vi "Init Test Group.vi"(8 "error in (no error)":errorcluster, 11 "Servo MSMT in":refnum<class "Servo MSMT.lvclass">) -> (0 "error out":errorcluster, 3 "Servo MSMT out":refnum<class "Servo MSMT.lvclass">)   [LabVIEW 2018, in "Servo MSMT.lvlib" / "Servo MSMT.lvclass"]
uses:
  Servo MSMT.lvclass
  Plugins/String Database.lvlibp/String Database.lvclass
  Plugins/Test Group Manager.lvlibp/Test Group Manager.lvclass
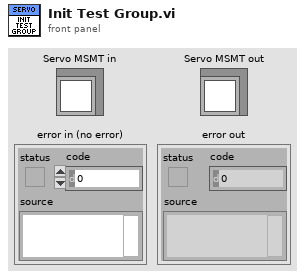
[diagram p1: front panel]
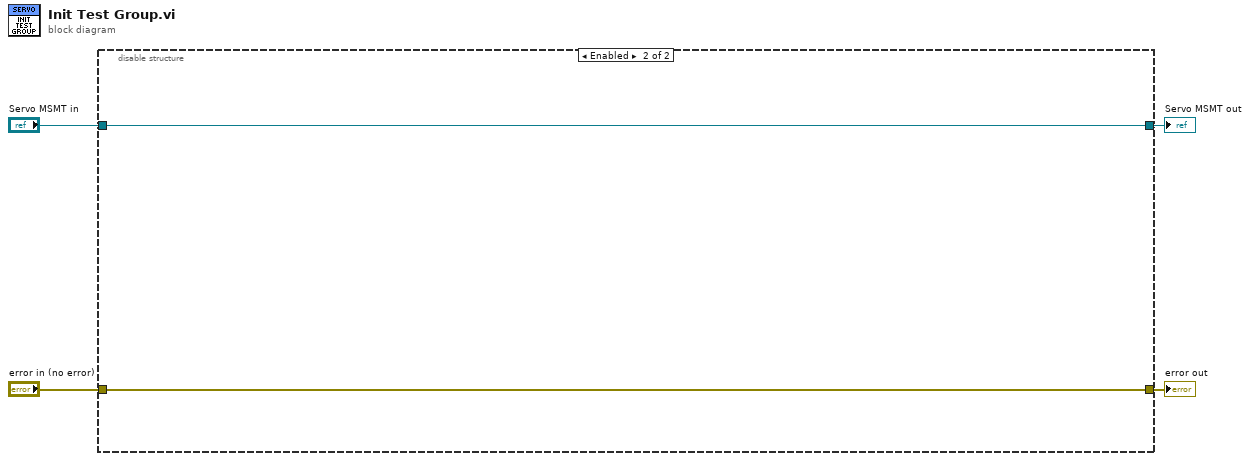
[diagram p0: block diagram]
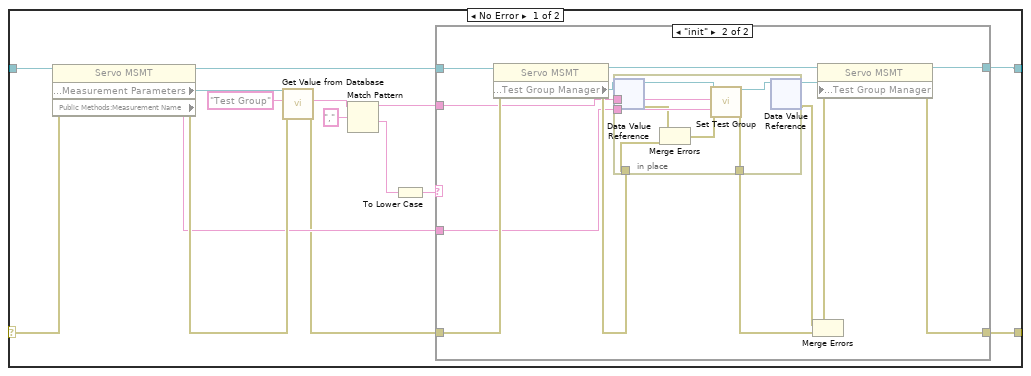
[diagram p3: hidden frame]
diagram:
  n1 = disable-structure shown="Enabled" {
    disable-tunnel: "error in (no error)" -> [w8 w49]
    disable-tunnel: [w7 w49] -> w3
    disable-tunnel: "Servo MSMT in" -> [w6 w50]
    disable-tunnel: [w5 w50] -> w1
    frame Disabled {
      n2 = case shown="Error" w8 {
        selector: w8 -> [w23 w48]
        tunnel: [w11 w48] -> w7
        tunnel: [w9 w47] -> w5
        tunnel: w6 -> [w22 w47]
        frame No Error {
          n3 = property class="Servo MSMT"(reference=w22, error in=w23) -> (reference out=w12:refnum<class "Servo MSMT.lvclass">, error out=w20:errorcluster, "Protected Methods:Measurement Parameters"=w21:refnum<class "String Database.lvclass">, "Public Methods:Measurement Name"=w13:string)
          n4 = call "Get Value from Database.vi"("error in (no error)"=w20, "Entry Name"="Test Group", "Message in"=w21) -> ("error out"=w10:errorcluster, "Entry Value"=w18:string)  [unwired: 5 in, 2 out]
          n5 = Match Pattern(string=w18, regular expression=",") -> (before substring=w14:string, after substring=w16:string)  [unwired: 1 in, 2 out]
          n6 = To Lower Case(string=w16) -> (all lower case string=w15:string)
          n7 = case shown="\"init\"" w15 {
            tunnel: w14 -> [_ w34]
            tunnel: w13 -> [_ w33]
            tunnel: w12 -> [w24 w38]
            tunnel: [w25 w32] -> w11
            tunnel: w10 -> [w25 w37]
            tunnel: [w24 w30] -> w9
            frame "False", Default {
            }
            frame "init" {
              n8 = property class="Servo MSMT"(reference=w38, error in=w37) -> (reference out=w31:refnum<class "Servo MSMT.lvclass">, error out=w36:errorcluster, "Protected Methods:Test Group Manager"=w29:refnum<data-value>)
              n9 = in-place {
                in-place-border: w36 -> [w40]
                in-place-border: [w46] -> w35
                in-place-border: w34 -> [w45]
                in-place-border: w33 -> [w44]
                n10 = in-place-dvr #1(w29) -> (w43:refnum<class "Test Group Manager.lvclass">, w41:errorcluster)
                n11 = Merge Errors(w41, w40) -> (w39:errorcluster)
                n12 = call "Set Test Group.vi"("Test Group Manager in"=w43, "Test Group Name"=w45, "Input Power"=w44, "error in (no error)"=w39) -> ("Test Group Manager out"=w42:refnum<class "Test Group Manager.lvclass">, "error out"=w46:errorcluster)  [unwired: 14 in]
                n13 = in-place-dvr #1(w42) -> (w28:refnum<data-value>, w26:errorcluster)
              }
              n14 = Merge Errors(w26, w35) -> (w27:errorcluster)
              n15 = property class="Servo MSMT"(reference=w31, error in=w27, "Protected Methods:Test Group Manager"=w28) -> (reference out=w30:refnum<class "Servo MSMT.lvclass">, error out=w32:errorcluster)
            }
          }
        }
        frame Error {
        }
      }
    }
    frame Enabled {
    }
  }
  "error out" <- w3
  "Servo MSMT out" <- w1
